vi "Write State DVR.vi"(8 "error in (no error)":errorcluster, 10 "State DVR":refnum<data-value>, 11 "Check Ozone Stability in":refnum<class "Check Ozone Stability.lvclass">) -> (0 "error out":errorcluster, 3 "Check Ozone Stability out":refnum<class "Check Ozone Stability.lvclass">)   [LabVIEW 2013, in "Check Ozone Stability.lvclass"]
uses:
  Check Ozone Stability.lvclass
  Data/cPAS Data.lvclass
  Check Ozone Stability.lvclass/Check Ozone Stability.ctl
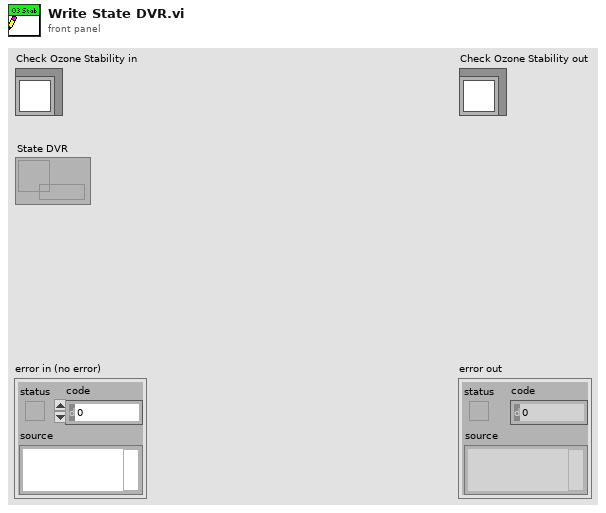
[diagram p1: front panel]
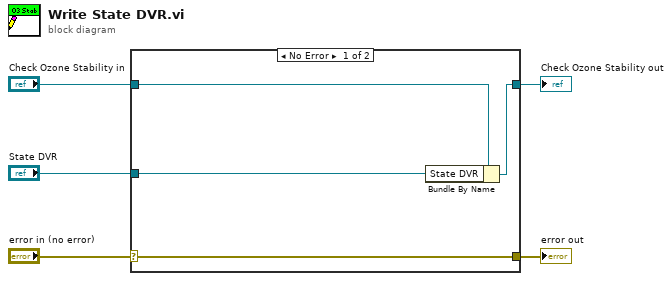
[diagram p0: block diagram]
diagram:
  n1 = case shown="No Error" "error in (no error)" {
    selector: "error in (no error)" -> [w9 w10]
    tunnel: [w9 w10] -> w4
    tunnel: [w7 w11] -> w2
    tunnel: "Check Ozone Stability in" -> [w8 w11]
    tunnel: "State DVR" -> [w6 _]
    frame No Error {
      n2 = Bundle By Name(cluster=w8, "State DVR"=w6) -> (w7:refnum<class "Check Ozone Stability.lvclass">)
    }
    frame Error {
    }
  }
  "error out" <- w4
  "Check Ozone Stability out" <- w2
